vi "Rio_Motion_Control.vi"(8 "Error In":errorcluster) -> (0 "Error Out":errorcluster)   [LabVIEW 2017]
doc: "This VI controls the X, Y and Theta axis given posiiton and angle inputs.\n\nWritten by Stefan Clarkson, Robin Moore & Thomas Quinn 26/02/18."
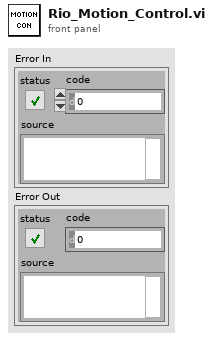
[diagram p1: front panel]
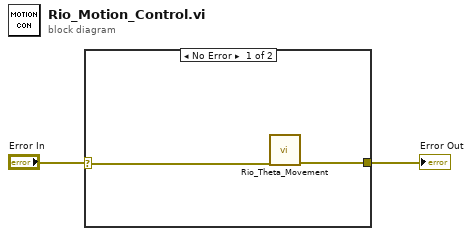
[diagram p0: block diagram]
diagram:
  n1 = case shown="No Error" "Error In" {
    selector: "Error In" -> [w4 w5]
    tunnel: [w3 w5] -> w1
    frame No Error {
      n2 = call "Rio_Theta_Movement.vi"("Error In"=w4) -> ("error out"=w3:errorcluster)  [unwired: 10 in]
    }
    frame Error {
    }
  }
  "Error Out" <- w1
